vi "Main.vi"() -> ()   [LabVIEW 2020]
uses:
  <vilib>/Utility/miscctls.llb/LVRectTypeDef.ctl
  <vilib>/UPVI/lvhdf5/group.llb/H5G_obj_t.ctl
  <vilib>/UPVI/lvhdf5/dataset.llb/LVH5D Operation.ctl
  <vilib>/Analysis/2dsp.llb/2D Convolution (DBL).vi
  <vilib>/Analysis/2dsp.llb/1D Convolution (DBL).vi
  <vilib>/UPVI/lvhdf5/utility.llb/Select HDF5 Dialog.vi
  <vilib>/UPVI/lvhdf5/utility.llb/Select HDF5 Dialog (Object Only).vi
  <vilib>/UPVI/lvhdf5/dataset.llb/Simple H5Dread (Variant).vi
  <vilib>/UPVI/lvhdf5/attribute.llb/Simple H5Aread (Variant).vi
  <vilib>/UPVI/lvhdf5/dataset.llb/Simple H5Dread.xnode
  <vilib>/UPVI/lvhdf5/library.llb/HDF5 Ref.ctl
  <vilib>/UPVI/lvhdf5/attribute.llb/Simple H5Aread.xnode
  <vilib>/UPVI/lvhdf5/file.llb/LVH5F Operation.ctl
  <vilib>/UPVI/lvhdf5/identifier.llb/Not an HDF5 Refnum Constant.vi
  <vilib>/UPVI/lvhdf5/dataset.llb/OpenCreateReplace Dataset.vi
  <vilib>/UPVI/lvhdf5/dataset.llb/H5Dget_space.vi
  <vilib>/UPVI/lvhdf5/dataspace.llb/H5Sget_simple_extent_dims.vi
  <vilib>/UPVI/lvhdf5/dataspace.llb/H5Sselect_hyperslab.vi
  <vilib>/UPVI/lvhdf5/dataset.llb/H5Dread (Variant).vi
  <vilib>/UPVI/lvhdf5/attribute.llb/private/LVH5AreadWDTAttrs.vi
  <vilib>/UPVI/lvhdf5/dataspace.llb/H5Sclose.vi
  <vilib>/Utility/error.llb/Error Cluster From Error Code.vi
  <vilib>/UPVI/lvhdf5/dataset.llb/H5Dclose.vi
  <vilib>/Analysis/NI_AALPro.lvlib
  <vilib>/UPVI/lvhdf5/utility.llb/Select HDF5 Dialog (File and Object).vi
panel:
  in  "Row Select":i32(slide) scale=0.0..8000.0
  out "Waveform Graph":dbl[](graph)
  in  "Clear Slot2":bool
  in  "Save Slot2":bool
  in  "Clear Slot1":bool
  in  "Save Slot1":bool
  in  "Apply Filter Bttn":bool
  in  "Image Correction and Control":enum32{"Gaussian Filter", "Matched Filter"}(tab)
  in  "Kernel Size":i32=3
  in  "sigma 2":i32=1
  in  "Kernel":dbl
  in  "sigma 3":dbl
  in  "Min Theta":i32=10
  in  "Max theta":i32=100
  in  "Theta Gap":i32=10
  out "Slot2 Image":picture caption="Slot 2 / Filtered Image"
  in  "Slot1 Image":picture caption="Slot 1 / Preview"
  in  "Data Filter Parameter Control":enum32{"Gaussian Filter", "Any New Filter"}(tab)
  in  "sigma":dbl=1.0
  in  "mean":dbl
  in  "Any New Filter":bool
  in  "Save Original Image Bttn":bool
  in  "Gaussian Filter":bool
  in  "Matched Filter":bool
  in  "RUN":bool
  out "TOF led":bool caption="Time of Flight Mode"
  out "Peak led":bool=TRUE caption="Peak Amplitude Mode"
  out "Progress":u8(slide) scale=0.0..100.0
  out "Time Steps":dbl
  out "Y Dim":dbl
  out "X Dim":dbl
  in  "Mode Selector Tab":T1(tab) caption="Mode Select"
  in  "Enable Threshold":bool=TRUE caption="Threshold"
  in  "Enable Window":bool=TRUE caption="Window"
  in  "Length":i32=2048
  in  "Window Start":i32 caption="Start Index"
  in  "Gate Threshold":dbl
  in  "No. Of layers":i32(slide)=2 min=2 max=2048 step=1 scale=2.0..500.0
  in  "Layer Gap":dbl=10.0
  in  "Layer no.":dbl caption="Layer Start"
  in  "Single Layer":bool
  in  "Slot 2 Copy":bool caption="Slot 2"
  in  "Slot 1 Copy":bool caption="Slot 1"
  in  "Clear Original Image":bool
  in  "Layer Selector Slider":i32(slide) caption="Layer Number" scale=0.0..195.0
  out "Original Picture":picture caption="Original"
  in  "Stop Bttn":bool
  out "File Loaded":bool
  in  "Open File Bttn":bool
  in  "File Path":path
  # "Load Image"
  # "The Filter will be applied on image in slot 1 and the result will be \ndisplayed in the slot 2."
  # "Data Analyzer"
  # "Note:\nKernel Size Must be Odd"
  # "Kernel Parameters:"
  # "Angle Parameters:"
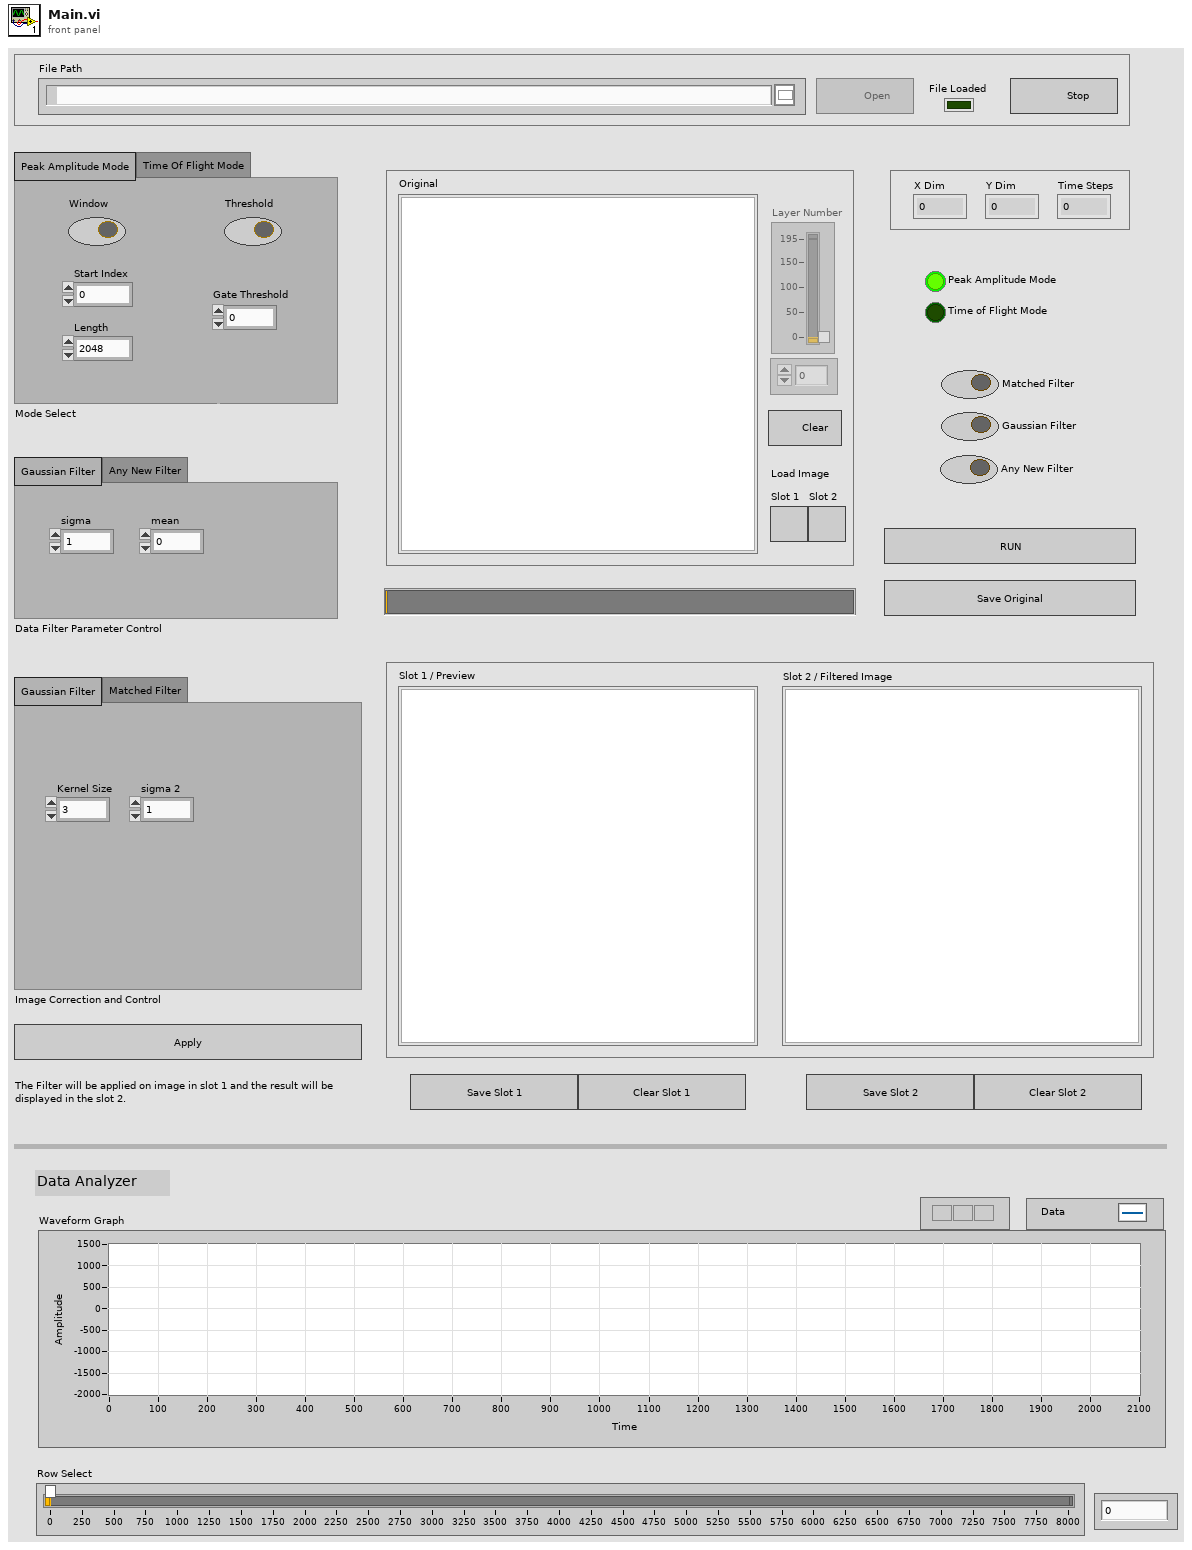
[diagram p1: front panel]
types:
  T1 = enum32{"Peak Amplitude Mode", "Time Of Flight Mode"}
  T2 = enum8{"Enabled", "Disabled", "Disabled and Grayed Out"}
  T3 = typedef "imagedata.ctl" = cluster{"image type":i32, "image depth":i32, "image":u8[], "mask":u8[], "colors":u32[], "Rectangle":cluster{"left":i16, "top":i16, "right":i16, "bottom":i16}}
  T4 = typedef "LVRectTypeDef.ctl" = cluster{"Left":i16, "Top":i16, "Right":i16, "Bottom":i16}
  T5 = cluster{"Behavior":enum32{"Invalid", "Default", "Floating", "Floating/Auto-Hide", "Modal"}, "Position":T4, "Center":bool, "Title":string}
  T6 = typedef "LVH5D Operation.ctl" = enum16{"open", "replace", "create", "open or create", "create or replace", "create or replace with confirmation"}
  T7 = typedef "LVH5F Operation.ctl" = enum16{"open", "open or create", "create or replace", "create or replace (with confirmation)", "create", "open (read only)"}
  T8 = typedef "H5G_obj_t.ctl" = i32
  T9 = cluster{"Object Types (any)":T8[], "Object Pattern":string}
  T10 = typedef "HDF5 Ref.ctl" = refnum<k1>
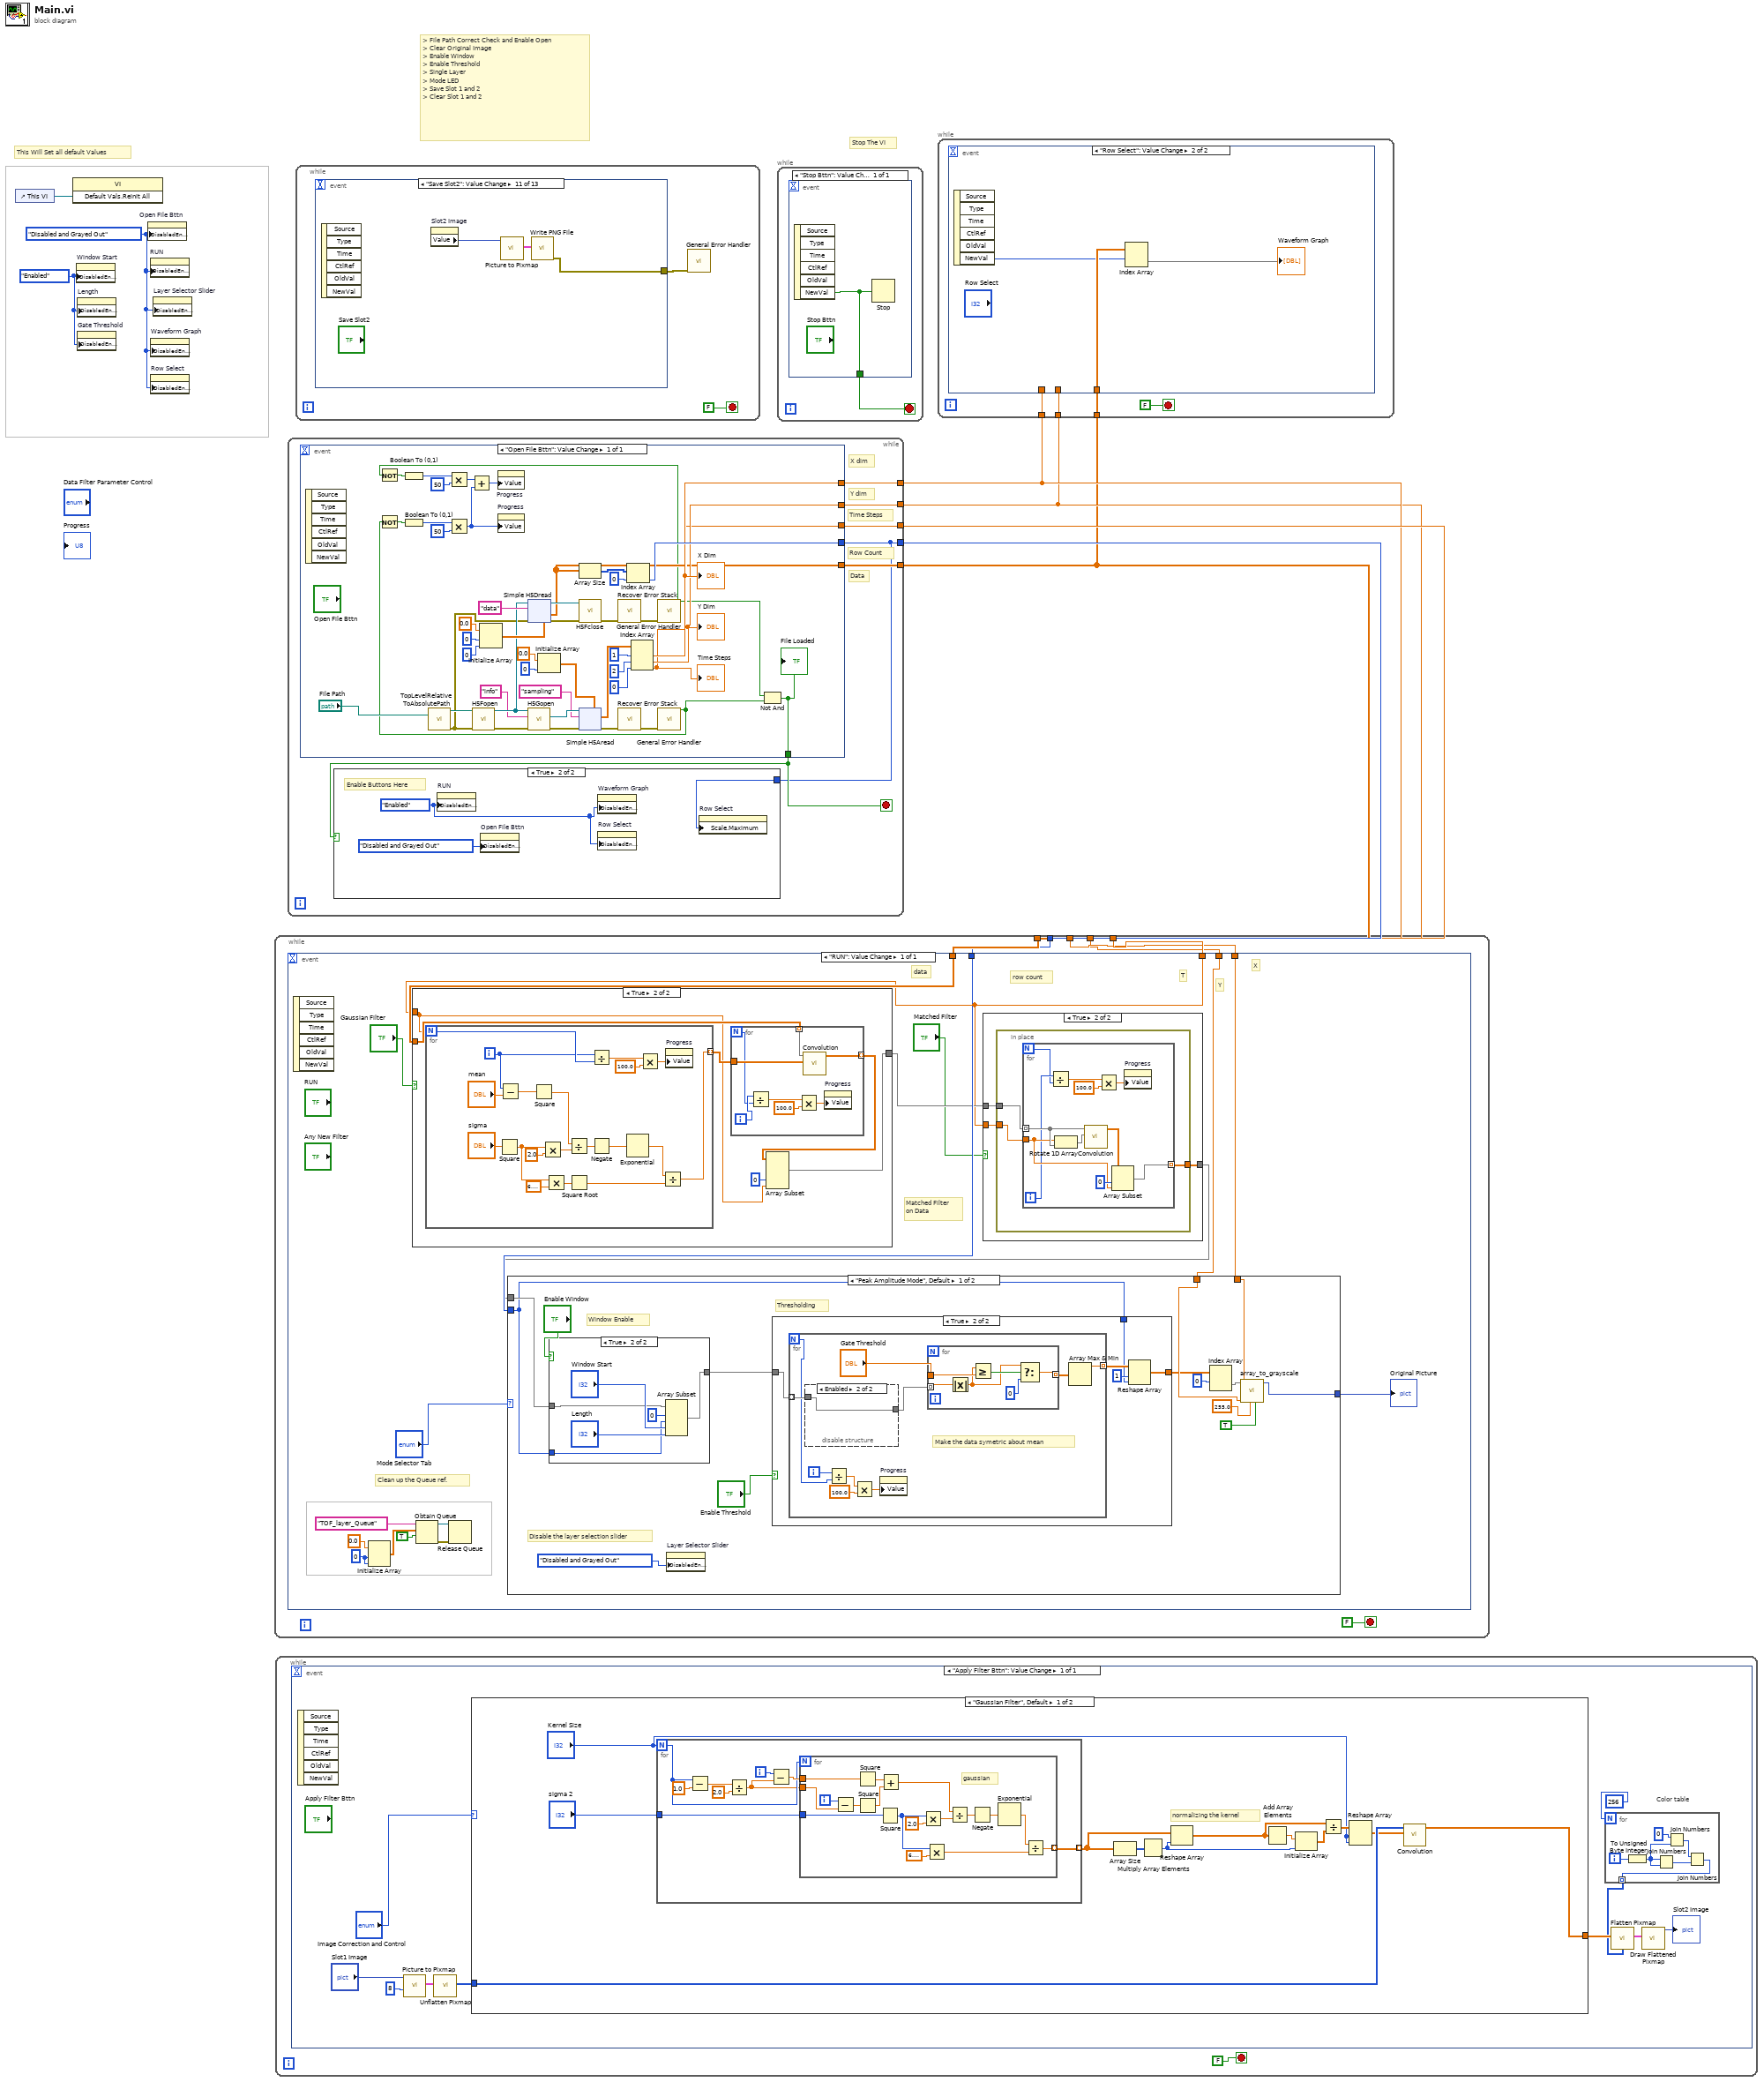
[diagram p0: block diagram]
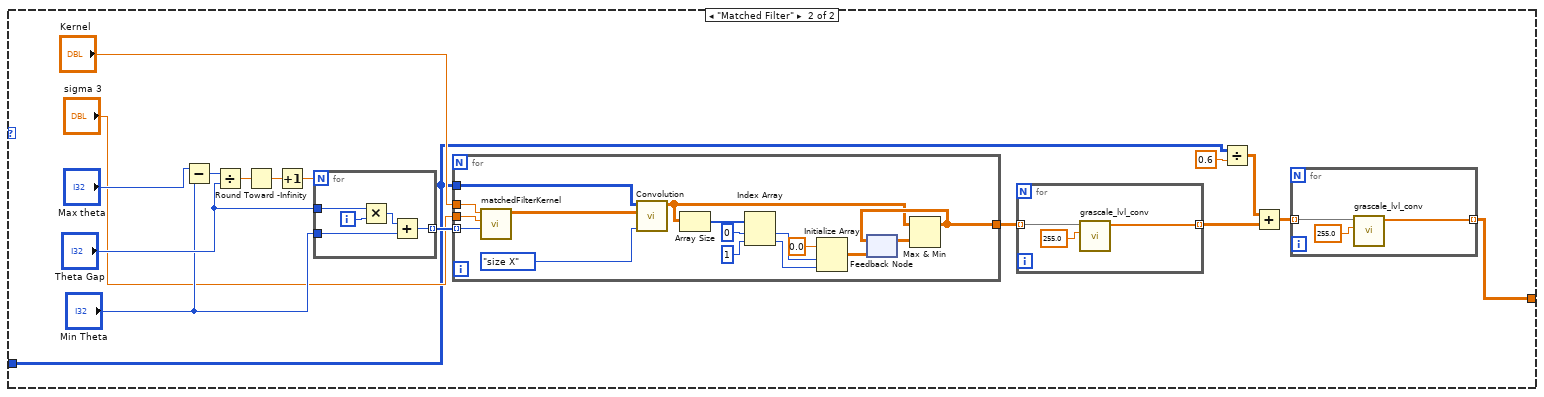
[diagram p2: hidden frame]
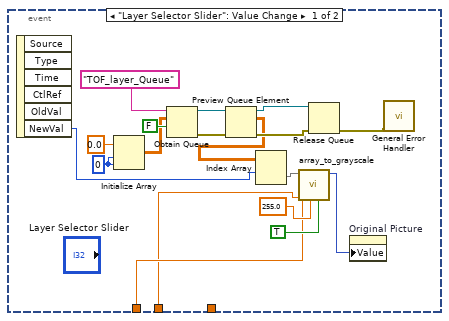
[diagram p3: hidden frame]
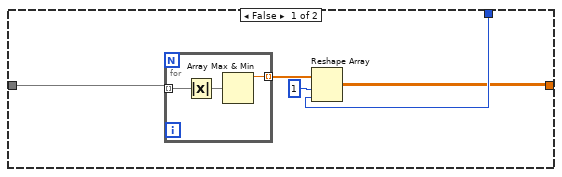
[diagram p6: hidden frame]
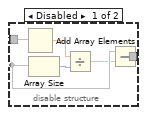
[diagram p7: hidden frame]
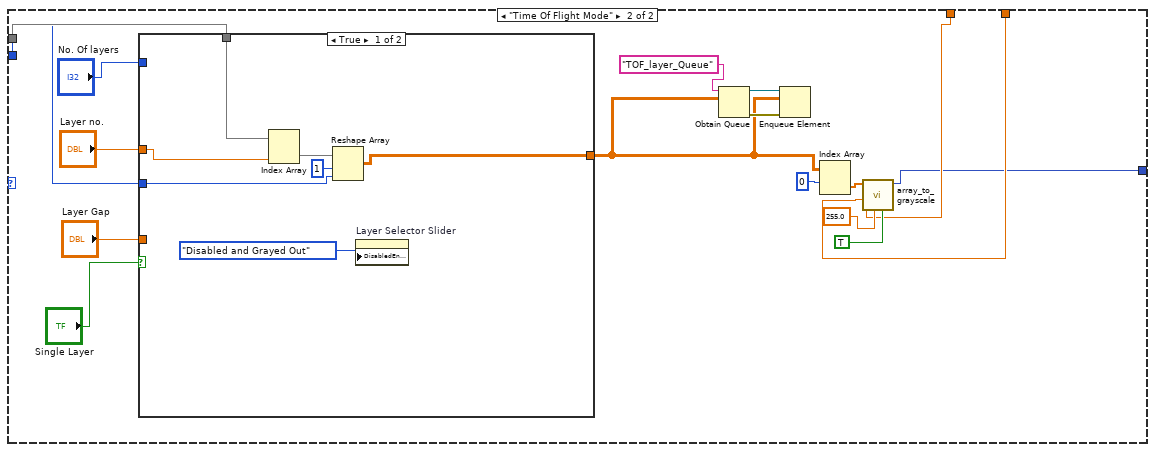
[diagram p9: hidden frame]
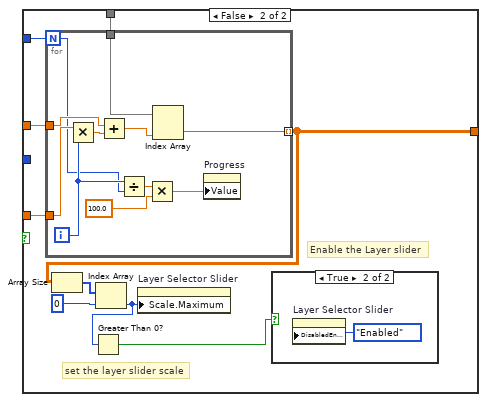
[diagram p10: hidden frame]
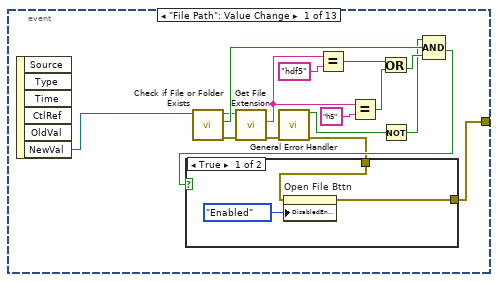
[diagram p12: hidden frame]
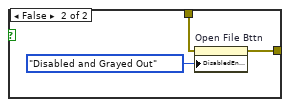
[diagram p13: hidden frame]
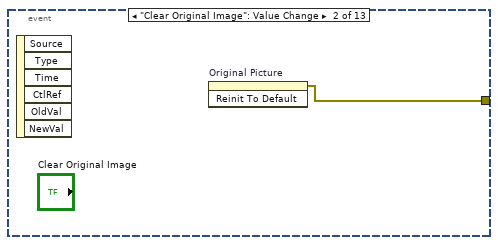
[diagram p14: hidden frame]
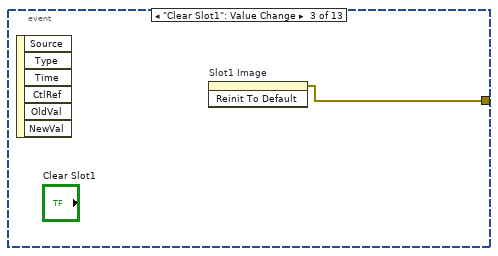
[diagram p15: hidden frame]
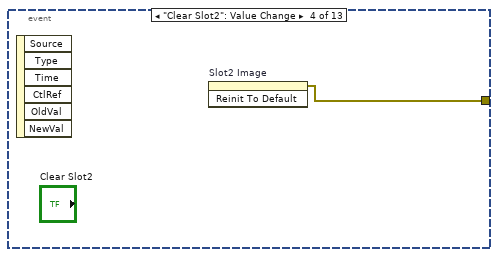
[diagram p16: hidden frame]
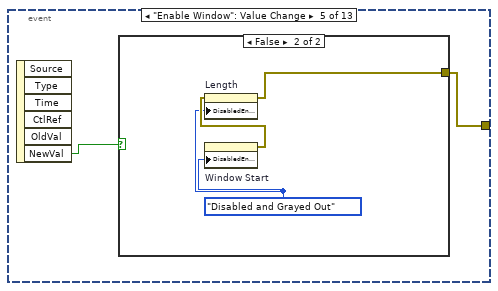
[diagram p17: hidden frame]
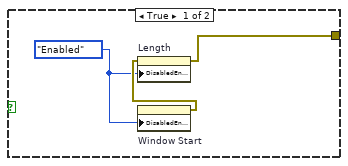
[diagram p18: hidden frame]
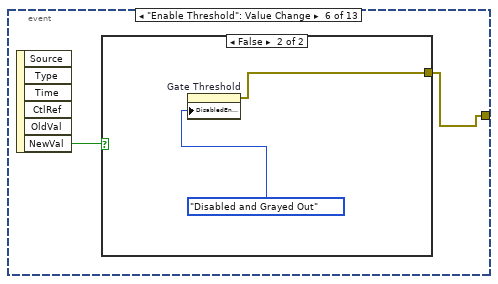
[diagram p19: hidden frame]
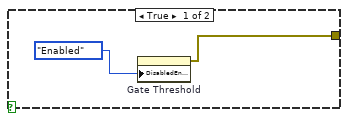
[diagram p20: hidden frame]
diagram:
  w5 = T2."Enabled" ("Disabled")
  w2 = T2."Disabled and Grayed Out" ("Disabled")
  # "This Will Set all default Values"
  # "> File Path Correct Check and Enable Open\n> Clear Original Image\n> Enable Window\n> Enable Threshold\n> Single Layer\n> Mode LED\n> Save Slot 1 and 2\n> Clear Slot 1 and 2"
  # "Stop The VI"
  n1 = control-ref of="This VI"() -> (w8:refnum<vi>)
  n2 = invoke class="VI" method="Default Vals.Reinit All"(reference=w8) -> ()  [unwired: 2 in, 3 out]
  n3 = property on="Window Start" class="DigNum (strict)"("DisabledEnum"=w5) -> ()  [unwired: 2 in, 2 out]
  n4 = property on="Length" class="DigNum (strict)"("DisabledEnum"=w5) -> ()  [unwired: 2 in, 2 out]
  n5 = property on="Gate Threshold" class="DigNum (strict)"("DisabledEnum"=w5) -> ()  [unwired: 2 in, 2 out]
  n6 = property on="Open File Bttn" class="Bool (strict)"("DisabledEnum"=w2) -> ()  [unwired: 2 in, 2 out]
  n7 = property on="RUN" class="Bool (strict)"("DisabledEnum"=w2) -> ()  [unwired: 2 in, 2 out]
  n8 = property on="Waveform Graph" class="WFGraph (strict)"("DisabledEnum"=w2) -> ()  [unwired: 2 in, 2 out]
  n9 = property on="Row Select" class="Slide (strict)"("DisabledEnum"=w2) -> ()  [unwired: 2 in, 2 out]
  n10 = property on="Layer Selector Slider" class="Slide (strict)"("DisabledEnum"=w2) -> ()  [unwired: 2 in, 2 out]
  n11 = while {
    stop <- FALSE stop-if-true
    n12 = event shown="[0] \"Apply Filter Bttn\": Value Change" {
      selector: _ -> [_]
      dyn-events: _ -> [_]
      timeout: _ -> [_]
      event "Apply Filter Bttn": Value Change {
        # "Color table"
        n13 = event-data() -> ()  [unwired: 1 in, 6 out]
        n14 = call <vilib>:"Picture to Pixmap.vi"("depth"=8, "picture"="Slot1 Image") -> ("image data"=w18:T3)  [unwired: 8 in, 1 out]
        n15 = call <vilib>:"Unflatten Pixmap.vi"("image data"=w18) -> ("8-bit pixmap"=w16:u8[][])  [unwired: 4 in, 6 out]
        n16 = case shown="\"Gaussian Filter\", Default" "Image Correction and Control" {
          tunnel: [w37 w69] -> w14
          tunnel: w16 -> [w36 w64]
          frame "Gaussian Filter", Default {
            # "normalizing the kernel"
            n17 = for {
              N: "Kernel Size" -> [w39]
              tunnel: "sigma 2" -> [w46]
              tunnel: [w45] -> w29 mode=indexing
              i -> [w43]
              n18 = Subtract(x=w39, y=1.0) -> (x-y=w40:dbl)
              n19 = Divide(x=w40, y=2.0) -> (x/y=w38:dbl)
              n20 = Subtract(x=w43, y=w38) -> (x-y=w44:dbl)
              n21 = for {
                N: w39 -> [_]
                tunnel: w44 -> [w49]
                tunnel: w46 -> [w48]
                tunnel: [w47] -> w45 mode=indexing
                tunnel: w38 -> [w62]
                i -> [w63]
                # "gaussian"
                n22 = Subtract(x=w63, y=w62) -> (x-y=w50:dbl)
                n23 = Square(x=w49) -> (x^2=w60:dbl)
                n24 = Square(x=w50) -> (x^2=w59:dbl)
                n25 = Square(x=w48) -> (x^2=w56:i32)
                n26 = Add(x=w60, y=w59) -> (x+y=w58:dbl)
                n27 = Multiply(x=w56, y=2.0) -> (x*y=w55:dbl)
                n28 = Multiply(x=w56, y=6.283185307179586) -> (x*y=w51:dbl)
                n29 = Divide(x=w58, y=w55) -> (x/y=w54:dbl)
                n30 = Negate(x=w54) -> (-x=w53:dbl)
                n31 = Exponential(1:w53) -> (0:w52:dbl)
                n32 = Divide(x=w52, y=w51) -> (x/y=w47:dbl)
              }
            }
            n33 = Array Size(array=w29) -> (size(s)=w33:i32[])
            n34 = Multiply Array Elements(1:w33) -> (0:w32:i32)
            n35 = Reshape Array(w29, w32) -> (w31:dbl[])
            n36 = Add Array Elements(numeric array=w31) -> (sum=w30:dbl)
            n37 = Initialize Array(w30, w32) -> (w34:dbl[])
            n38 = Divide(x=w31, y=w34) -> (x/y=w35:dbl[])
            n39 = Reshape Array(w35, "Kernel Size", "Kernel Size") -> (w26:dbl[][])
            n40 = call-poly <vilib>:"Convolution.vi"("Y"=w26, "X"=w36) -> ("X * Y"=w37:dbl[][])  [unwired: 8 in, 1 out]
          }
          frame "Matched Filter" {
            n41 = Subtract(x="Max theta", y="Min Theta") -> (x-y=w75:i32)
            n42 = Divide(x=w75, y="Theta Gap") -> (x/y=w77:dbl)
            n43 = Round Toward -Infinity(1:w77) -> (0:w78:dbl)
            n44 = Increment(x=w78) -> (x+1=w79:dbl)
            n45 = for {
              N: w79 -> [_]
              tunnel: "Theta Gap" -> [w90]
              tunnel: "Min Theta" -> [w88]
              tunnel: [w87] -> w80 mode=indexing
              i -> [w91]
              n46 = Multiply(x=w90, y=w91) -> (x*y=w89:i32)
              n47 = Add(x=w89, y=w88) -> (x+y=w87:i32)
            }
            n48 = for {
              tunnel: "Kernel" -> [w107]
              tunnel: "sigma 3" -> [w106]
              tunnel: w80 -> [w105] mode=indexing
              tunnel: w64 -> [w94]
              tunnel: [w102] -> w70
              n49 = call "matchedFilterKernel.vi"("theta"=w105, "sigma"=w106, "L"=w107) -> ("Array"=w93:dbl[][])  [unwired: 8 in]
              n50 = call-poly <vilib>:"Convolution.vi"("output size"=enum32{"full", "size X", "compact"}."size X", "Y"=w93, "X"=w94) -> ("X * Y"=w92:dbl[][])  [unwired: 7 in, 1 out]
              n51 = Array Size(array=w92) -> (size(s)=w100:i32[])
              n52 = Index Array(array=w100, index #1=0 ("index"), index #2=1 ("index")) -> (element #1=w98:i32, element #2=w97:i32)
              n53 = Initialize Array(0.0 ("element"), w98, w97) -> (w96:dbl[][])
              n54 = feedback #1(w96) -> (w104:dbl[][])
              n55 = Max & Min(x=w92, y=w104) -> (max(x,y)=w102:dbl[][])  [unwired: 1 out]
              n56 = feedback-in #1(w102) -> ()
            }
            n57 = for {
              tunnel: w70 -> [w85] mode=indexing
              tunnel: [w84] -> w67 mode=indexing
              n58 = call "grascale_lvl_conv.vi"("max level"=255.0 ("y"), "Array in"=w85) -> ("Array out"=w84:dbl[])  [unwired: 9 in]
            }
            n59 = Divide(x=w64, y=0.6) -> (x/y=w65:dbl[][])
            n60 = Add(x=w65, y=w67) -> (x+y=w68:dbl[][])
            n61 = for {
              tunnel: w68 -> [w82] mode=indexing
              tunnel: [w81] -> w69 mode=indexing
              n62 = call "grascale_lvl_conv.vi"("max level"=255.0 ("y"), "Array in"=w82) -> ("Array out"=w81:dbl[])  [unwired: 9 in]
            }
          }
        }
        n63 = for {
          N: 256 -> [_]
          tunnel: [w20] -> w10 mode=indexing
          i -> [w25]
          n64 = To Unsigned Byte Integer(number=w25) -> (unsigned 8bit integer=w24:u8)
          n65 = Join Numbers(hi=w24, lo=w24) -> ((hi.lo)=w21:u16)
          n66 = Join Numbers(hi=u8 0, lo=w24) -> ((hi.lo)=w22:u16)
          n67 = Join Numbers(hi=w22, lo=w21) -> ((hi.lo)=w20:u32)
        }
        n68 = call <vilib>:"Flatten Pixmap.vi"("colors"=w10, "8-bit pixmap"=w14) -> ("image data"=w15:T3)  [unwired: 9 in]
        n69 = call <vilib>:"Draw Flattened Pixmap.vi"("image data"=w15) -> ("new picture"=→"Slot2 Image":picture)  [unwired: 8 in]
      }
    }
  }
  n70 = while {
    tunnel: [w112] -> w4
    tunnel: [w111] -> w3
    tunnel: [w110] -> w6
    tunnel: [w108] -> w7
    tunnel: [w109] -> w1
    stop <- w113 stop-if-true
    # "Data"
    # "Row Count"
    # "Time Steps"
    # "Y dim"
    # "X dim"
    n71 = event shown="[0] \"Open File Bttn\": Value Change" {
      selector: _ -> [_]
      dyn-events: _ -> [_]
      timeout: _ -> [_]
      tunnel: [w134] -> w108
      tunnel: [w133] -> w112
      tunnel: [w132] -> w111
      tunnel: [w131] -> w110
      tunnel: [w118] -> w113
      tunnel: [w130] -> w109
      event "Open File Bttn": Value Change {
        n72 = event-data() -> ()  [unwired: 1 in, 6 out]
        n73 = call "TopLevelRelativeToAbsolutePath.vi"("Path Relative to Top Level VI"="File Path") -> ("error out"=w119:errorcluster, "Absolute path"=w152:path)  [unwired: 9 in]
        n74 = call <vilib>:"H5Fopen.vi"("error in (no error)"=w119, "path"=w152) -> ("error out"=w147:errorcluster, "HDF5 Ref out"=w150:T10)  [unwired: 6 in]
        n75 = Initialize Array(0.0 ("element"), 0 ("dimension size"), 0 ("dimension size")) -> (w151:dbl[][])
        n76 = call <vilib>:"H5Gopen.vi"("error in (no error)"=w147, "Name"="info" ("Dataset Path"), "HDF5 Ref"=w150) -> ("error out"=w144:errorcluster, "HDF5 Group Ref"=w146:T10)  [unwired: 4 in, 1 out]
        n77 = xnode "Simple H5Dread"("Dataset Path"="data", "error in (no error)"=w119, "HDF5 Path or Ref"=w150, "Data"=w151) -> ("HDF5 Ref out"=w156:T10, "error out"=w155:errorcluster, "Data out"=w130:dbl[][])  [unwired: 1 out]
        n78 = Initialize Array(0.0 ("element"), 0 ("dimension size")) -> (w140:dbl[])
        n79 = Array Size(array=w130) -> (size(s)=w154:i32[])
        n80 = call <vilib>:"H5Fclose.vi"("error in (no error)"=w155, "HDF5 Ref"=w156) -> ("error out"=w161:errorcluster)  [unwired: 7 in]
        n81 = xnode "Simple H5Aread"("HDF5 Ref"=w146, "Name"="sampling", "error in (no error)"=w144, "Type"=w140) -> ("error out"=w143:errorcluster, "Value"=w139:dbl[])  [unwired: 1 out]
        n82 = call <vilib>:"Recover Error Stack.vi"("error in (no error)"=w161) -> ("error out"=w162:errorcluster)  [unwired: 5 in, 3 out]
        n83 = call <vilib>:"Recover Error Stack.vi"("error in (no error)"=w143) -> ("error out"=w148:errorcluster)  [unwired: 5 in, 3 out]
        n84 = Index Array(array=w154, index=0) -> (element=w134:i32)
        n85 = Index Array(array=w139, index #1=1 ("index"), index #2=2 ("index"), index #3=0 ("index")) -> (element #1=w133:dbl, element #2=w132:dbl, element #3=w131:dbl)
        "X Dim" <- w133
        "Y Dim" <- w132
        "Time Steps" <- w131
        n86 = call <vilib>:"General Error Handler.vi"("error in (no error)"=w162) -> ("error?"=w128:bool)  [unwired: 10 in, 4 out]
        n87 = Not(x=w128) -> (.not. x?=w129:bool)
        n88 = Boolean To (0,1)(Boolean=w129) -> (0, 1=w125:i16)
        n89 = Multiply(x=w125, y=i16 50) -> (x*y=w123:i16)
        n90 = call <vilib>:"General Error Handler.vi"("error in (no error)"=w148) -> ("error?"=w126:bool)  [unwired: 10 in, 4 out]
        n91 = Not(x=w126) -> (.not. x?=w127:bool)
        n92 = Boolean To (0,1)(Boolean=w127) -> (0, 1=w120:i16)
        n93 = Multiply(x=w120, y=i16 50) -> (x*y=w117:i16)
        n94 = Add(x=w123, y=w117) -> (x+y=w122:i16)
        n95 = property on="Progress" class="Slide (strict)"("Value"=w122) -> ()  [unwired: 2 in, 2 out]
        n96 = property on="Progress" class="Slide (strict)"("Value"=w117) -> ()  [unwired: 2 in, 2 out]
        n97 = Not And(1:w126, 2:w128) -> (0:w118:bool)
        "File Loaded" <- w118
      }
    }
    n98 = case shown="True" w113 {
      tunnel: w108 -> [_ w114]
      frame False {
      }
      frame True {
        w115 = T2."Enabled" ("Disabled")
        # "Enable Buttons Here"
        n99 = property on="RUN" class="Bool (strict)"("DisabledEnum"=w115) -> ()  [unwired: 2 in, 2 out]
        n100 = property on="Open File Bttn" class="Bool (strict)"("DisabledEnum"=T2."Disabled and Grayed Out" ("Disabled")) -> ()  [unwired: 2 in, 2 out]
        n101 = property on="Waveform Graph" class="WFGraph (strict)"("DisabledEnum"=w115) -> ()  [unwired: 2 in, 2 out]
        n102 = property on="Row Select" class="Slide (strict)"("DisabledEnum"=w115) -> ()  [unwired: 2 in, 2 out]
        n103 = property on="Row Select" class="Slide (strict)"("Scale.Maximum"=w114) -> ()  [unwired: 2 in, 2 out]
      }
    }
  }
  n104 = while {
    tunnel: w1 -> [w509]
    tunnel: w7 -> [w508]
    tunnel: w6 -> [w506]
    tunnel: w3 -> [w504]
    tunnel: w4 -> [w505]
    stop <- FALSE stop-if-true
    n105 = event shown="[0] \"RUN\": Value Change" {
      selector: _ -> [_]
      dyn-events: _ -> [_]
      timeout: _ -> [_]
      tunnel: w509 -> [w514]
      tunnel: w508 -> [w527]
      tunnel: w506 -> [w512]
      tunnel: w504 -> [w525]
      tunnel: w505 -> [w524]
      event "RUN": Value Change {
        w518 = 0 ("dimension size")
        # "Matched Filter\non Data"
        # "Clean up the Queue ref."
        # "data"
        # "row count"
        # "T"
        # "Y"
        # "X"
        n106 = event-data() -> ()  [unwired: 1 in, 6 out]
        n107 = Initialize Array(0.0 ("element"), w518, w518) -> (w516:dbl[][])
        n108 = case shown="True" "Gaussian Filter" {
          tunnel: w514 -> [w546 w552]
          tunnel: [w546 w549] -> w513
          tunnel: w512 -> [_ w547]
          frame False {
          }
          frame True {
            n109 = for {
              N: w547 -> [w562]
              tunnel: [w566] -> w551 mode=indexing
              i -> [w561]
              n110 = Square(x="sigma") -> (x^2=w570:dbl)
              n111 = Subtract(x=w561, y="mean") -> (x-y=w577:dbl)
              n112 = Square(x=w577) -> (x^2=w575:dbl)
              n113 = Multiply(x=w570, y=2.0) -> (x*y=w574:dbl)
              n114 = Multiply(x=w570, y=6.283185307179586) -> (x*y=w569:dbl)
              n115 = Divide(x=w575, y=w574) -> (x/y=w573:dbl)
              n116 = Square Root(x=w569) -> (sqrt(x)=w567:dbl)
              n117 = Divide(x=w561, y=w562) -> (x/y=w565:dbl)
              n118 = Negate(x=w573) -> (-x=w572:dbl)
              n119 = Exponential(1:w572) -> (0:w568:dbl)
              n120 = Multiply(x=w565, y=100.0) -> (x*y=w563:dbl)
              n121 = Divide(x=w568, y=w567) -> (x/y=w566:dbl)
              n122 = property on="Progress" class="Slide (strict)"("Value"=w563) -> ()  [unwired: 2 in, 2 out]
            }
            n123 = for {
              N -> [w553]
              tunnel: w552 -> [w560] mode=indexing
              tunnel: w551 -> [w559]
              tunnel: [w558] -> w550 mode=indexing
              i -> [w554]
              n124 = Divide(x=w554, y=w553) -> (x/y=w555:dbl)
              n125 = Multiply(x=w555, y=100.0) -> (x*y=w557:dbl)
              n126 = call-poly <vilib>:"Convolution.vi"("Y"=w559, "X"=w560) -> ("X * Y"=w558:dbl[])  [unwired: 8 in, 1 out]
              n127 = property on="Progress" class="Slide (strict)"("Value"=w557) -> ()  [unwired: 2 in, 2 out]
            }
            n128 = Array Subset(array=w550, index (col)=0 ("index"), length (col)=w547) -> (w549:dbl[][])  [unwired: 2 in]
          }
        }
        n129 = Obtain Queue(name (unnamed)="TOF_layer_Queue", element data type=w516, create if not found? (T)=TRUE) -> (queue out=w522:refnum<queue>, error out=w520:errorcluster)  [unwired: 2 in, 1 out]
        n130 = Release Queue(queue=w522, error in (no error)=w520) -> ()  [unwired: 1 in, 3 out]
        n131 = case shown="True" "Matched Filter" {
          tunnel: [w528 w531] -> w511
          tunnel: w513 -> [w528 w530]
          tunnel: w512 -> [_ w529]
          frame False {
          }
          frame True {
            n132 = in-place {
              in-place-border: [w534] -> w531
              in-place-border: w530 -> [w533]
              in-place-border: w529 -> [w532]
              n133 = for {
                N -> [w535]
                tunnel: [w542] -> w534 mode=indexing
                tunnel: w533 -> [w541] mode=indexing
                tunnel: w532 -> [w540]
                i -> [w536]
                n134 = Divide(x=w536, y=w535) -> (x/y=w537:dbl)
                n135 = Rotate 1D Array(1:w541, 2:w540) -> (0:w545:dbl[])
                n136 = call-poly <vilib>:"Convolution.vi"("Y"=w545, "X"=w541) -> ("X * Y"=w544:dbl[])  [unwired: 8 in, 1 out]
                n137 = Multiply(x=w537, y=100.0) -> (x*y=w539:dbl)
                n138 = Array Subset(array=w544, index=0, length=w540) -> (w542:dbl[])
                n139 = property on="Progress" class="Slide (strict)"("Value"=w539) -> ()  [unwired: 2 in, 2 out]
              }
            }
          }
        }
        n140 = case shown="\"Peak Amplitude Mode\", Default" "Mode Selector Tab" {
          tunnel: w511 -> [w592 w649]
          tunnel: w527 -> [w589 w647]
          tunnel: w525 -> [w584 w639]
          tunnel: w524 -> [w581 w640]
          tunnel: [w582 w638] -> w523
          frame "Peak Amplitude Mode", Default {
            # "Disable the layer selection slider"
            # "Thresholding"
            # "Window Enable"
            n141 = case shown="True" "Enable Window" {
              tunnel: [w629 w632] -> w591
              tunnel: w592 -> [w629 w631]
              tunnel: w589 -> [_ w630]
              frame False {
              }
              frame True {
                n142 = Array Subset(array=w631, index (row)=0 ("index"), length (row)=w630, index (col)="Window Start", length (col)="Length") -> (w632:dbl[][])
              }
            }
            n143 = property on="Layer Selector Slider" class="Slide (strict)"("DisabledEnum"=T2."Disabled and Grayed Out" ("Disabled")) -> ()  [unwired: 2 in, 2 out]
            n144 = case shown="True" "Enable Threshold" {
              tunnel: w591 -> [w598 w606]
              tunnel: [w594 w604] -> w583
              tunnel: w589 -> [w596 w602]
              frame False {
                n145 = for {
                  tunnel: w598 -> [w601] mode=indexing
                  tunnel: [w599] -> w595 mode=indexing
                  n146 = Absolute Value(x=w601) -> (abs(x)=w600:dbl[])
                  n147 = Array Max & Min(array=w600) -> (max value=w599:dbl)  [unwired: 3 out]
                }
                n148 = Reshape Array(w595, 1 ("dimension size"), w596) -> (w594:dbl[][])
              }
              frame True {
                n149 = for {
                  N -> [w607]
                  tunnel: w606 -> [w616] mode=indexing
                  tunnel: [w608] -> w605 mode=indexing
                  i -> [w612]
                  # "Make the data symetric about mean"
                  n150 = disable-structure shown="Enabled" {
                    disable-tunnel: w616 -> [w619 w622]
                    disable-tunnel: [w617 w622] -> w615
                    frame Disabled {
                      n151 = Add Array Elements(numeric array=w619) -> (sum=w621:dbl)
                      n152 = Array Size(array=w619) -> (size(s)=w620:i32)
                      n153 = Divide(x=w621, y=w620) -> (x/y=w618:dbl)
                      n154 = Subtract(x=w619, y=w618) -> (x-y=w617:dbl[])
                    }
                    frame Enabled {
                    }
                  }
                  n155 = Divide(x=w612, y=w607) -> (x/y=w611:dbl)
                  n156 = Multiply(x=w611, y=100.0) -> (x*y=w609:dbl)
                  n157 = property on="Progress" class="Slide (strict)"("Value"=w609) -> ()  [unwired: 2 in, 2 out]
                  n158 = for {
                    tunnel: w615 -> [w628] mode=indexing
                    tunnel: "Gate Threshold" -> [w627]
                    tunnel: [w623] -> w613 mode=indexing
                    n159 = Absolute Value(x=w628) -> (abs(x)=w625:dbl)
                    n160 = Greater Or Equal?(x=w625, y=w627) -> (x >= y?=w626:bool)
                    n161 = Select(t=w625, s=w626, f=0) -> (s? t:f=w623:dbl)
                  }
                  n162 = Array Max & Min(array=w613) -> (max value=w608:dbl)  [unwired: 3 out]
                }
                n163 = Reshape Array(w605, 1 ("dimension size"), w602) -> (w604:dbl[][])
              }
            }
            n164 = Index Array(array=w583, index (row)=0) -> (element=w585:dbl[])  [unwired: 1 in]
            n165 = call "array_to_grayscale.vi"("Y Flip"=TRUE, "max level"=255.0, "Y Dim"=w584, "X Dim"=w581, "Input"=w585) -> ("picture"=w582:picture)  [unwired: 5 in, 1 out]
          }
          frame "Time Of Flight Mode" {
            n166 = case shown="True" "Single Layer" {
              tunnel: "Layer Gap" -> [_ w668]
              tunnel: "No. Of layers" -> [_ w667]
              tunnel: "Layer no." -> [w658 w666]
              tunnel: w649 -> [w659 w665]
              tunnel: [w656 w662] -> w636
              tunnel: w647 -> [w654 _]
              frame True {
                n167 = Index Array(array=w659, index (col)=w658) -> (element=w657:dbl[])  [unwired: 1 in]
                n168 = Reshape Array(w657, 1 ("dimension size"), w654) -> (w656:dbl[][])
                n169 = property on="Layer Selector Slider" class="Slide (strict)"("DisabledEnum"=T2."Disabled and Grayed Out" ("Disabled")) -> ()  [unwired: 2 in, 2 out]
              }
              frame False {
                # "set the layer slider scale"
                # "Enable the Layer slider"
                n170 = for {
                  N: w667 -> [w673]
                  tunnel: w666 -> [w680]
                  tunnel: w668 -> [w679]
                  tunnel: w665 -> [w677]
                  tunnel: [w675] -> w662 mode=indexing
                  i -> [w674]
                  n171 = Multiply(x=w679, y=w674) -> (x*y=w678:dbl)
                  n172 = Add(x=w680, y=w678) -> (x+y=w676:dbl)
                  n173 = Divide(x=w674, y=w673) -> (x/y=w672:dbl)
                  n174 = Multiply(x=w672, y=100.0) -> (x*y=w670:dbl)
                  n175 = Index Array(array=w677, index (col)=w676) -> (element=w675:dbl[])  [unwired: 1 in]
                  n176 = property on="Progress" class="Slide (strict)"("Value"=w670) -> ()  [unwired: 2 in, 2 out]
                }
                n177 = Array Size(array=w662) -> (size(s)=w663:i32[])
                n178 = Index Array(array=w663, index=0) -> (element=w661:i32)
                n179 = Greater Than 0?(x=w661) -> (x > 0?=w660:bool)
                n180 = property on="Layer Selector Slider" class="Slide (strict)"("Scale.Maximum"=w661) -> ()  [unwired: 2 in, 2 out]
                n181 = case shown="True" w660 {
                  frame False {
                  }
                  frame True {
                    n182 = property on="Layer Selector Slider" class="Slide (strict)"("DisabledEnum"=T2."Enabled" ("Disabled")) -> ()  [unwired: 2 in, 2 out]
                  }
                }
              }
            }
            n183 = Obtain Queue(name (unnamed)="TOF_layer_Queue", element data type=w636) -> (queue out=w645:refnum<queue>, error out=w637:errorcluster)  [unwired: 3 in, 1 out]
            n184 = Enqueue Element(queue=w645, element=w636, error in (no error)=w637) -> ()  [unwired: 1 in, 3 out]
            n185 = Index Array(array=w636, index (row)=0) -> (element=w641:dbl[])  [unwired: 1 in]
            n186 = call "array_to_grayscale.vi"("Y Flip"=TRUE, "max level"=255.0, "Y Dim"=w639, "X Dim"=w640, "Input"=w641) -> ("picture"=w638:picture)  [unwired: 5 in, 1 out]
          }
        }
        "Original Picture" <- w523
      }
    }
  }
  n187 = while {
    stop <- FALSE stop-if-true
    n188 = event shown="[10] \"Save Slot2\": Value Change" {
      selector: _ -> [_ _ _ _ _ _ _ _ _ _ _ _ _]
      dyn-events: _ -> [_ _ _ _ _ _ _ _ _ _ _ _ _]
      timeout: _ -> [_ _ _ _ _ _ _ _ _ _ _ _ _]
      tunnel: [w683 w705 w706 w707 w708 w717 w723 _ w737 w740 w743 w746 w749] -> w681
      event "File Path": Value Change {
        n189 = event-data() -> ("NewVal"=w685:path)  [unwired: 1 in, 5 out]
        n190 = call <vilib>:"Check if File or Folder Exists.vi"("path"=w685) -> ("error out"=w686:errorcluster, "file or folder exists?"=w696:bool, "dup path"=w688:path)  [unwired: 8 in]
        n191 = call <vilib>:"Get File Extension.vi"("error in (no error)"=w686, "file"=w688) -> ("error out"=w687:errorcluster, "lowercase file extension"=w691:string)  [unwired: 5 in, 3 out]
        n192 = call <vilib>:"General Error Handler.vi"("error in (no error)"=w687) -> ("error?"=w694:bool, "error out"=w684:errorcluster)  [unwired: 10 in, 3 out]
        n193 = Equal?(x=w691, y="hdf5") -> (x = y?=w693:bool)
        n194 = Equal?(x=w691, y="h5") -> (x = y?=w692:bool)
        n195 = Or(x=w693, y=w692) -> (x .or. y?=w697:bool)
        n196 = Not(x=w694) -> (.not. x?=w695:bool)
        n197 = Compound Arithmetic op=AND(w695, w696, w697) -> (w698:bool)
        n198 = case shown="True" w698 {
          tunnel: w684 -> [w700 w703]
          tunnel: [w699 w702] -> w683
          frame True {
            n199 = property on="Open File Bttn" class="Bool (strict)"(error in=w700, "DisabledEnum"=T2."Enabled" ("Disabled")) -> (error out=w699:errorcluster)  [unwired: 1 in, 1 out]
          }
          frame False {
            n200 = property on="Open File Bttn" class="Bool (strict)"(error in=w703, "DisabledEnum"=T2."Disabled and Grayed Out" ("Disabled")) -> (error out=w702:errorcluster)  [unwired: 1 in, 1 out]
          }
        }
      }
      event "Clear Original Image": Value Change {
        n201 = event-data() -> ()  [unwired: 1 in, 6 out]
        n202 = invoke on="Original Picture" class="Pict" method="Reinit To Default"() -> (error out=w705:errorcluster)  [unwired: 3 in, 2 out]
      }
      event "Clear Slot1": Value Change {
        n203 = event-data() -> ()  [unwired: 1 in, 6 out]
        n204 = invoke on="Slot1 Image" class="Pict" method="Reinit To Default"() -> (error out=w706:errorcluster)  [unwired: 3 in, 2 out]
      }
      event "Clear Slot2": Value Change {
        n205 = event-data() -> ()  [unwired: 1 in, 6 out]
        n206 = invoke on="Slot2 Image" class="Pict" method="Reinit To Default"() -> (error out=w707:errorcluster)  [unwired: 3 in, 2 out]
      }
      event "Enable Window": Value Change {
        n207 = event-data() -> ("NewVal"=w709:bool)  [unwired: 1 in, 5 out]
        n208 = case shown="False" w709 {
          tunnel: [w712 w715] -> w708
          frame True {
            w710 = T2."Enabled" ("Disabled")
            n209 = property on="Window Start" class="DigNum (strict)"("DisabledEnum"=w710) -> (error out=w711:errorcluster)  [unwired: 2 in, 1 out]
            n210 = property on="Length" class="DigNum (strict)"(error in=w711, "DisabledEnum"=w710) -> (error out=w712:errorcluster)  [unwired: 1 in, 1 out]
          }
          frame False {
            w713 = T2."Disabled and Grayed Out" ("Disabled")
            n211 = property on="Window Start" class="DigNum (strict)"("DisabledEnum"=w713) -> (error out=w714:errorcluster)  [unwired: 2 in, 1 out]
            n212 = property on="Length" class="DigNum (strict)"(error in=w714, "DisabledEnum"=w713) -> (error out=w715:errorcluster)  [unwired: 1 in, 1 out]
          }
        }
      }
      event "Enable Threshold": Value Change {
        n213 = event-data() -> ("NewVal"=w716:bool)  [unwired: 1 in, 5 out]
        n214 = case shown="False" w716 {
          tunnel: [w719 w721] -> w717
          frame True {
            n215 = property on="Gate Threshold" class="DigNum (strict)"("DisabledEnum"=T2."Enabled" ("Disabled")) -> (error out=w719:errorcluster)  [unwired: 2 in, 1 out]
          }
          frame False {
            n216 = property on="Gate Threshold" class="DigNum (strict)"("DisabledEnum"=T2."Disabled and Grayed Out" ("Disabled")) -> (error out=w721:errorcluster)  [unwired: 2 in, 1 out]
          }
        }
      }
      event "Single Layer": Value Change {
        n217 = event-data() -> ("NewVal"=w722:bool)  [unwired: 1 in, 5 out]
        n218 = case shown="False" w722 {
          tunnel: [w725 w728] -> w723
          frame True {
            w724 = T2."Disabled and Grayed Out" ("Disabled")
            n219 = property on="Layer Gap" class="DigNum (strict)"("DisabledEnum"=w724) -> (error out=w726:errorcluster)  [unwired: 2 in, 1 out]
            n220 = property on="No. Of layers" class="Slide (strict)"(error in=w726, "DisabledEnum"=w724) -> (error out=w725:errorcluster)  [unwired: 1 in, 1 out]
          }
          frame False {
            w727 = T2."Enabled" ("Disabled")
            n221 = property on="Layer Gap" class="DigNum (strict)"("DisabledEnum"=w727) -> (error out=w729:errorcluster)  [unwired: 2 in, 1 out]
            n222 = property on="No. Of layers" class="Slide (strict)"(error in=w729, "DisabledEnum"=w727) -> (error out=w728:errorcluster)  [unwired: 1 in, 1 out]
          }
        }
      }
      event "Mode Selector Tab": Value Change {
        n223 = event-data() -> ("NewVal"=w732:T1)  [unwired: 1 in, 5 out]
        n224 = case shown="\"Peak Amplitude Mode\", Default" w732 {
          tunnel: [TRUE FALSE] -> w731
          tunnel: [FALSE TRUE] -> w730
          frame "Peak Amplitude Mode", Default {
          }
          frame "Time Of Flight Mode" {
          }
        }
        "Peak led" <- w731
        "TOF led" <- w730
      }
      event "Save Original Image Bttn": Value Change {
        n225 = event-data() -> ()  [unwired: 1 in, 6 out]
        n226 = property on="Original Picture" class="Pict"() -> ("Value"=w739:picture)  [unwired: 2 in, 2 out]
        n227 = call <vilib>:"Picture to Pixmap.vi"("picture"=w739) -> ("image data"=w738:T3)  [unwired: 9 in, 1 out]
        n228 = call <vilib>:"Write PNG File.vi"("image data"=w738) -> ("error out"=w737:errorcluster)  [unwired: 9 in, 1 out]
      }
      event "Save Slot1": Value Change {
        n229 = event-data() -> ()  [unwired: 1 in, 6 out]
        n230 = property on="Slot1 Image" class="Pict"() -> ("Value"=w742:picture)  [unwired: 2 in, 2 out]
        n231 = call <vilib>:"Picture to Pixmap.vi"("picture"=w742) -> ("image data"=w741:T3)  [unwired: 9 in, 1 out]
        n232 = call <vilib>:"Write PNG File.vi"("image data"=w741) -> ("error out"=w740:errorcluster)  [unwired: 9 in, 1 out]
      }
      event "Save Slot2": Value Change {
        n233 = event-data() -> ()  [unwired: 1 in, 6 out]
        n234 = property on="Slot2 Image" class="Pict"() -> ("Value"=w745:picture)  [unwired: 2 in, 2 out]
        n235 = call <vilib>:"Picture to Pixmap.vi"("picture"=w745) -> ("image data"=w744:T3)  [unwired: 9 in, 1 out]
        n236 = call <vilib>:"Write PNG File.vi"("image data"=w744) -> ("error out"=w743:errorcluster)  [unwired: 9 in, 1 out]
      }
      event "Slot 1 Copy": Value Change {
        n237 = event-data() -> ()  [unwired: 1 in, 6 out]
        n238 = property on="Original Picture" class="Pict"() -> (error out=w747:errorcluster, "Value"=w748:picture)  [unwired: 2 in, 1 out]
        n239 = property on="Slot1 Image" class="Pict"(error in=w747, "Value"=w748) -> (error out=w746:errorcluster)  [unwired: 1 in, 1 out]
      }
      event "Slot 2 Copy": Value Change {
        n240 = event-data() -> ()  [unwired: 1 in, 6 out]
        n241 = property on="Original Picture" class="Pict"() -> (error out=w750:errorcluster, "Value"=w751:picture)  [unwired: 2 in, 1 out]
        n242 = property on="Slot2 Image" class="Pict"(error in=w750, "Value"=w751) -> (error out=w749:errorcluster)  [unwired: 1 in, 1 out]
      }
    }
    n243 = call <vilib>:"General Error Handler.vi"("error in (no error)"=w681) -> ()  [unwired: 10 in, 5 out]
  }
  n244 = while {
    stop <- w752 stop-if-true
    n245 = event shown="[0] \"Stop Bttn\": Value Change" {
      selector: _ -> [_]
      dyn-events: _ -> [_]
      timeout: _ -> [_]
      tunnel: [w753] -> w752
      event "Stop Bttn": Value Change {
        n246 = event-data() -> ("NewVal"=w753:bool)  [unwired: 1 in, 5 out]
        n247 = Stop(stop? (T)=w753) -> ()
      }
    }
  }
  n248 = while {
    tunnel: w4 -> [w756]
    tunnel: w3 -> [w755]
    tunnel: w1 -> [w754]
    stop <- FALSE stop-if-true
    n249 = event shown="[1] \"Row Select\": Value Change" {
      selector: _ -> [_ _]
      dyn-events: _ -> [_ _]
      timeout: _ -> [_ _]
      tunnel: w756 -> [w760 _]
      tunnel: w755 -> [w759 _]
      tunnel: w754 -> [_ w778]
      event "Layer Selector Slider": Value Change {
        w765 = 0 ("dimension size")
        n250 = event-data() -> ("NewVal"=w761:i32)  [unwired: 1 in, 5 out]
        n251 = Initialize Array(0.0 ("element"), w765, w765) -> (w763:dbl[][])
        n252 = Obtain Queue(name (unnamed)="TOF_layer_Queue", element data type=w763, create if not found? (T)=FALSE) -> (queue out=w767:refnum<queue>, error out=w766:errorcluster)  [unwired: 2 in, 1 out]
        n253 = Preview Queue Element(queue=w767, error in (no error)=w766) -> (queue out=w774:refnum<queue>, element=w771:dbl[][], error out=w775:errorcluster)  [unwired: 1 in, 1 out]
        n254 = Index Array(array=w771, index (row)=w761) -> (element=w770:dbl[])  [unwired: 1 in]
        n255 = call "array_to_grayscale.vi"("Y Flip"=TRUE, "max level"=255.0, "Y Dim"=w759, "X Dim"=w760, "Input"=w770) -> ("picture"=w772:picture)  [unwired: 5 in, 1 out]
        n256 = Release Queue(queue=w774, error in (no error)=w775) -> (error out=w758:errorcluster)  [unwired: 1 in, 2 out]
        n257 = property on="Original Picture" class="Pict"("Value"=w772) -> ()  [unwired: 2 in, 2 out]
        n258 = call <vilib>:"General Error Handler.vi"("error in (no error)"=w758) -> ()  [unwired: 10 in, 5 out]
      }
      event "Row Select": Value Change {
        n259 = event-data() -> ("NewVal"=w777:i32)  [unwired: 1 in, 5 out]
        n260 = Index Array(array=w778, index (row)=w777) -> (element=→"Waveform Graph":dbl[])  [unwired: 1 in]
      }
    }
  }
